vi "MAC_ColonToHex.vi"(11 "MAC Address (colon notation)":string) -> (3 "MAC Address (hex string)":string)   [LabVIEW 2014, in "hse-network.lvlib"]
doc: "(v0.2.1b; 2017-08-14 16:44)\n\n\n\n____\nHAMPEL SOFTWARE ENGINEERING v0.7.0 (2018-07-16 18:12)"
uses:
  hse-network.lvlib
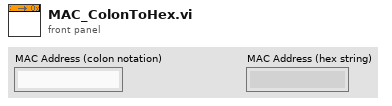
[diagram p1: front panel]
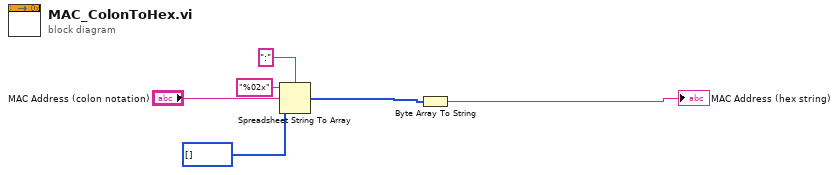
[diagram p0: block diagram]
diagram:
  n1 = Spreadsheet String To Array(delimiter (Tab)=":", format string="%02x", spreadsheet string="MAC Address (colon notation)", array type (2D Dbl)=u8[] [] ("Array 2")) -> (array=w2:u8[])
  n2 = Byte Array To String(unsigned byte array=w2) -> (string=→"MAC Address (hex string)":string)
